vi "模拟输入_保存.vi"() -> ()   [LabVIEW 2013]
doc: "This example demonstrates how to acquire a continuous data."
uses:
  <userlib>/ArtDAQ/_SubVI/ArtDAQ_CreateAIVoltageChan.vi
  <userlib>/ArtDAQ/_SubVI/ArtDAQ_CfgSampClkTiming.vi
  <userlib>/ArtDAQ/_SubVI/ArtDAQ_CfgDigEdgeStartTrig.vi
  <userlib>/ArtDAQ/_SubVI/ArtDAQ_CfgAnlgEdgeStartTrig.vi
  <userlib>/ArtDAQ/_SubVI/ArtDAQ_CfgAnlgWindowStartTrig.vi
  <userlib>/ArtDAQ/_SubVI/ArtDAQ_Read Analog DBL NChan NSamp.vi
panel:
  in  "文件路径":path=path "C:/Users/Administrator/Desktop/Data"
  in  "触发模式":enum32{"无触发", "数字边沿", "模拟边沿", "模拟窗"}(tab)
  in  "触发源":string="/Dev1/PFI1"
  in  "触发边沿":i32(ring)=10280 items=["上升"=10280, "下降"=10171]
  in  "触发电平(V)":dbl
  in  "触发源":string(combo)="Dev1/ai0"
  in  "斜率":i32(ring)=10280 items=["上升"=10280, "下降"=10171]
  in  "触发条件":i32(ring)=10163 items=["进入窗"=10163, "离开窗"=10208]
  in  "窗顶部":dbl=0.5
  in  "窗底部":dbl
  in  "触发源":string(combo)="Dev1/ai0"
  in  "停止":bool
  out "Waveform":dbl[][](graph)
  in  "采样频率":dbl=10000.0 format="%#_13g"
  in  "每通道采样点数":i32=1000
  in  "接地方式":i32(ring)=10083 items=["默认"=-1, "单端"=10083, "非参考单端"=10078, "差分"=10106, "伪差分"=12529]
  in  "最小值(V)":dbl=-10.0 format="%#_13g"
  in  "最大值(V)":dbl=10.0 format="%#_13g"
  in  "物理通道":string(combo)="Dev1/ai0"
  out "错误":errorcluster
  # "通道属性"
  # "定时"
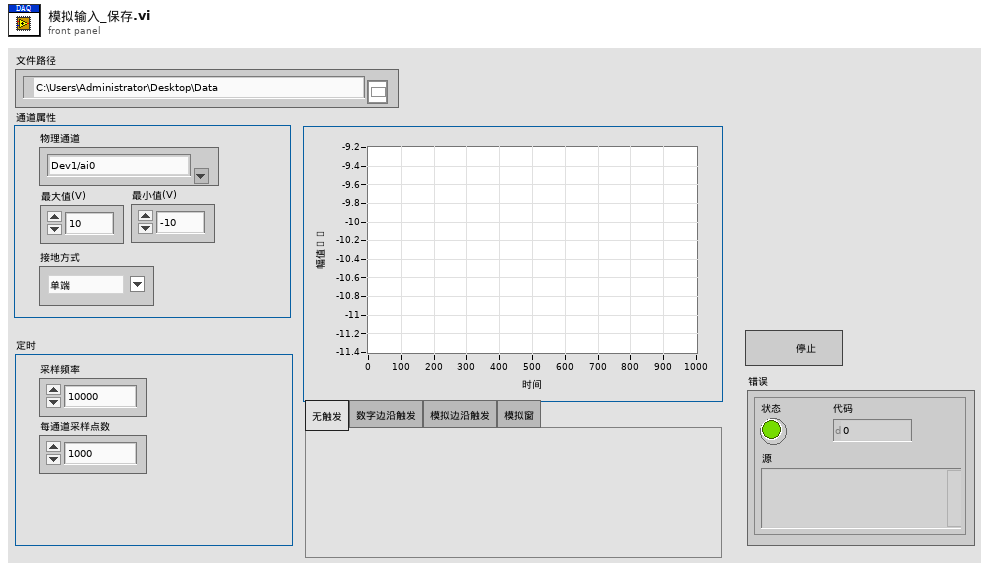
[diagram p1: front panel]
types:
  T1 = enum16{"open", "open or create", "create or replace", "create", "open (read-only)"}
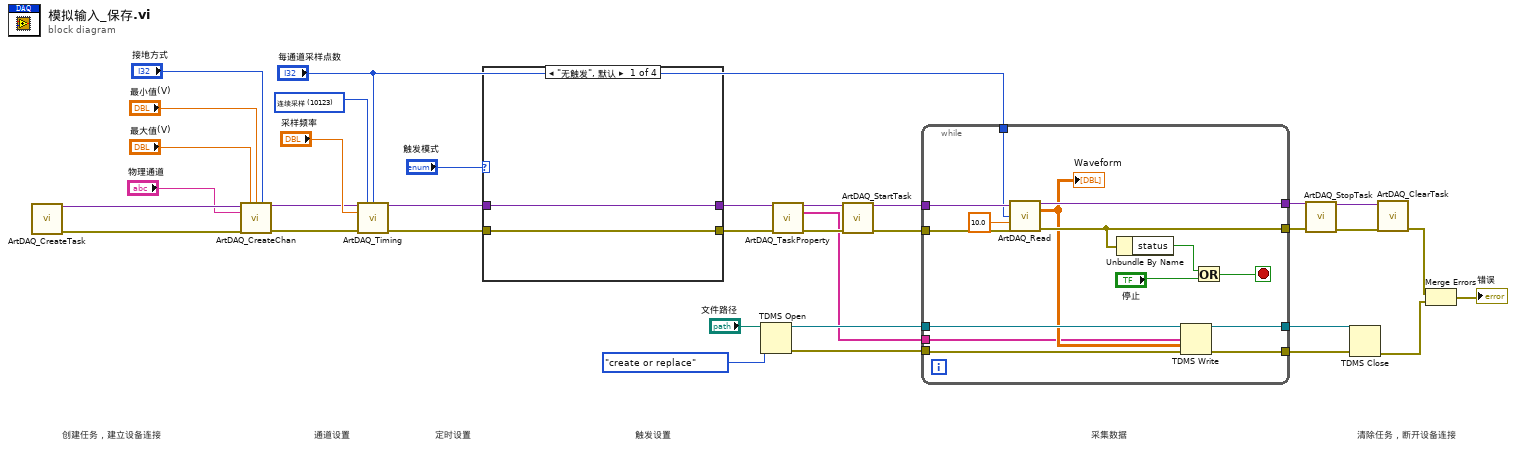
[diagram p0: block diagram]
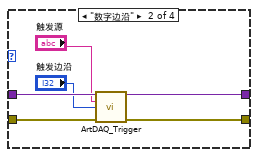
[diagram p2: hidden frame]
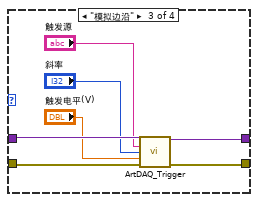
[diagram p3: hidden frame]
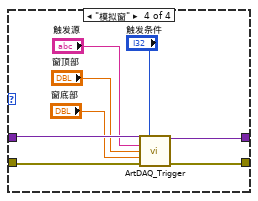
[diagram p4: hidden frame]
diagram:
  w16 = 10123 items=["有限点采样"=10178, "连续采样"=10123] ("SampleMode")
  # "清除任务，断开设备连接"
  # "采集数据"
  # "触发设置"
  # "定时设置"
  # "通道设置"
  # "创建任务，建立设备连接"
  n1 = call <userlib>:"ArtDAQ_CreateTask.vi"() -> ("任务句柄"=w25:variant, "错误输出"=w34:errorcluster)  [unwired: 14 in]
  n2 = call-poly <userlib>:"ArtDAQ_CreateChan.vi"("任务句柄"=w25, "最大值"="最大值(V)", "最小值"="最小值(V)", "接线端配置"="接地方式", "物理通道"="物理通道", "错误输入"=w34) -> ("任务句柄"=w17:variant, "错误输出"=w30:errorcluster)  [unwired: 8 in]
  n3 = call-poly <userlib>:"ArtDAQ_Timing.vi"("任务句柄"=w17, "采样模式"=w16, "每通道采样数"="每通道采样点数", "采样率"="采样频率", "错误输入"=w30) -> ("任务句柄"=w19:variant, "错误输出"=w18:errorcluster)  [unwired: 9 in]
  n4 = case shown="\"无触发\", 默认" "触发模式" {
    tunnel: w19 -> [w36 w42 w49 w57]
    tunnel: [w36 w41 w48 w56] -> w5
    tunnel: w18 -> [w35 w39 w46 w54]
    tunnel: [w35 w40 w47 w55] -> w2
    frame "无触发", Default {
    }
    frame "数字边沿" {
      n5 = call-poly <userlib>:"ArtDAQ_Trigger.vi"("任务句柄"=w42, "触发源"="触发源", "边沿"="触发边沿", "错误输入"=w39) -> ("任务句柄"=w41:variant, "错误输出"=w40:errorcluster)  [unwired: 10 in]
    }
    frame "模拟边沿" {
      n6 = call-poly <userlib>:"ArtDAQ_Trigger.vi"("任务句柄"=w49, "触发源"="触发源", "斜率"="斜率", "触发电平"="触发电平(V)", "错误输入"=w46) -> ("任务句柄"=w48:variant, "错误输出"=w47:errorcluster)  [unwired: 9 in]
    }
    frame "模拟窗" {
      n7 = call-poly <userlib>:"ArtDAQ_Trigger.vi"("任务句柄"=w57, "触发条件"="触发条件", "触发源"="触发源", "窗顶部"="窗顶部", "窗底部"="窗底部", "错误输入"=w54) -> ("任务句柄"=w56:variant, "错误输出"=w55:errorcluster)  [unwired: 8 in]
    }
  }
  n8 = TDMS Open(10:T1."create or replace" ("操作(0:open)"), 11:"文件路径") -> (0:w6:errorcluster, 3:w7:refnum<k34>)  [unwired: 5 in]
  n9 = call-poly <userlib>:"ArtDAQ_TaskProperty.vi"("任务句柄"=w5, "错误输入"=w2) -> ("任务句柄"=w4:variant, "通道名称"=w1:string[], "错误输出"=w3:errorcluster)  [unwired: 11 in]
  n10 = call <userlib>:"ArtDAQ_StartTask.vi"("任务句柄"=w4, "错误输入"=w3) -> ("任务句柄"=w28:variant, "错误输出"=w27:errorcluster)  [unwired: 12 in]
  n11 = while {
    tunnel: w28 -> [w72]
    tunnel: w27 -> [w71]
    tunnel: "每通道采样点数" -> [w70]
    tunnel: [w68] -> w24
    tunnel: [w67] -> w23
    tunnel: w7 -> [w63]
    tunnel: w6 -> [w62]
    tunnel: [w60] -> w13
    tunnel: [w59] -> w12
    tunnel: w1 -> [w58]
    stop <- w65 stop-if-true
    n12 = call-poly <userlib>:"ArtDAQ_Read.vi"("任务句柄"=w72, "每通道采样数"=w70, "超时s"=10.0 ("Timeout"), "错误输入"=w71) -> ("任务句柄"=w68:variant, "数据"=w61:dbl[][], "错误输出"=w67:errorcluster)  [unwired: 8 in, 1 out]
    "Waveform" <- w61
    n13 = Unbundle By Name(w67) -> ("status"=w66:bool)
    n14 = TDMS Write(0:w63, 7:w58, 9:w61, 11:w62) -> (4:w60:refnum<k34>, 15:w59:errorcluster)  [unwired: 2 in, 2 out]
    n15 = Or(x=w66, y="停止") -> (x .or. y?=w65:bool)
  }
  n16 = call <userlib>:"ArtDAQ_StopTask.vi"("任务句柄"=w24, "错误输入"=w23) -> ("任务句柄"=w22:variant, "错误输出"=w21:errorcluster)  [unwired: 12 in]
  n17 = TDMS Close(8:w12, 11:w13) -> (0:w11:errorcluster)  [unwired: 1 out]
  n18 = call <userlib>:"ArtDAQ_ClearTask.vi"("任务句柄"=w22, "错误输入"=w21) -> ("错误输出"=w10:errorcluster)  [unwired: 13 in]
  n19 = Merge Errors(w10, w11) -> (→"错误":errorcluster)
